vi "most basic edge detection.vi"(10 "falling edge":bool, 11 "pulse":bool) -> (3 "edge detected":bool)   [LabVIEW 2018]
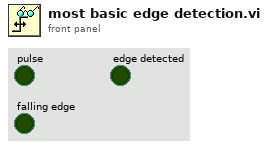
[diagram p1: front panel]
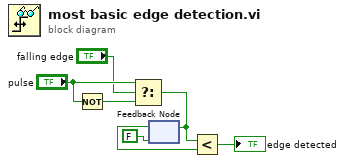
[diagram p0: block diagram]
diagram:
  n1 = Not(x="pulse") -> (.not. x?=w3:bool)
  n2 = Select(t="pulse", s="falling edge", f=w3) -> (s? t:f=w4:bool)
  n3 = feedback #1(FALSE ("filteredState")) -> (w6:bool)
  n4 = feedback-in #1(w4) -> ()
  n5 = Less?(x=w4, y=w6) -> (x < y?=→"edge detected":bool)
